vi "ControlSubMIMO.vi"(0 "AxisForceSample":dbl[](array[numeric]), 1 "Command":dbl[](array[numeric]), 3 "Angel":bool[](array[boolean]), 4 "AngleSample":dbl[](array[numeric]), 5 "TorqueSample":dbl[](array[numeric]), 6 "Torque":bool[](array[boolean]), 8 "syn-error":dbl[](array[numeric]), 11 "ChannelSetArray":T1[](array[typedef]) {"Enable" items=["不使能", "使能"]; "Wave" items=["0指令", "正弦波", "方波", "三角波", "常值", "波形数据", "白噪声", "正弦扫频", "梯度加载", "VMIC"]; "ChannelType" items=["标准波形跟踪"=1, "扫频测试"=2, "消除多余力"=3, "梯度加载"=4, "载荷谱跟踪"=5, "模拟输入跟踪"=9]; "ChannelStatus" items=["通道关", "位置通道", "加载通道"]}, 12 "dt":dbl) -> (14 "ControlOutput":dbl[](array[numeric]))   [LabVIEW 2020]
uses:
  ChannelCommand.ctl
  Control 1.ctl
  WaveType.ctl
  MoterEnable.ctl
panel:
  in  "ControlPara":dbl[][](array[numeric])
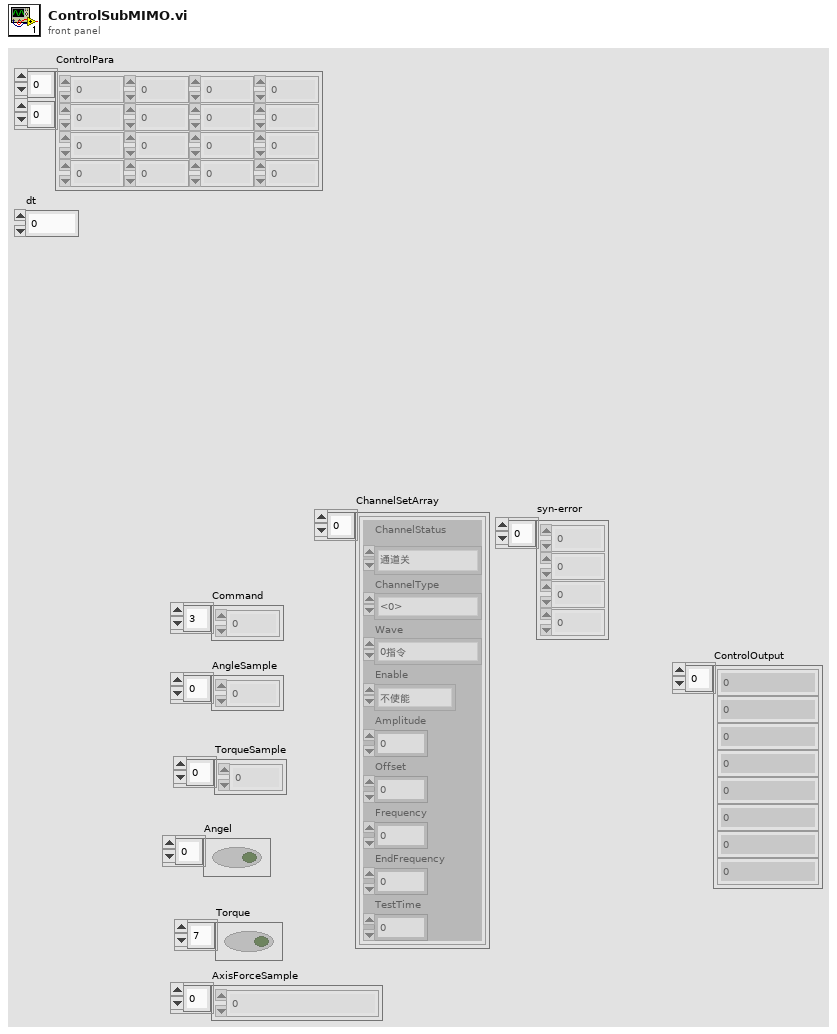
[diagram p1: front panel]
types:
  T1 = typedef "ChannelCommand.ctl" = cluster{"ChannelStatus":T2, "ChannelType":i32, "Wave":T3, "Enable":T4, "Amplitude":dbl, "Offset":dbl, "Frequency":dbl, "EndFrequency":dbl, "TestTime":dbl}
  T2 = typedef "Control 1.ctl" = i32
  T3 = typedef "WaveType.ctl" = i32
  T4 = typedef "MoterEnable.ctl" = u16
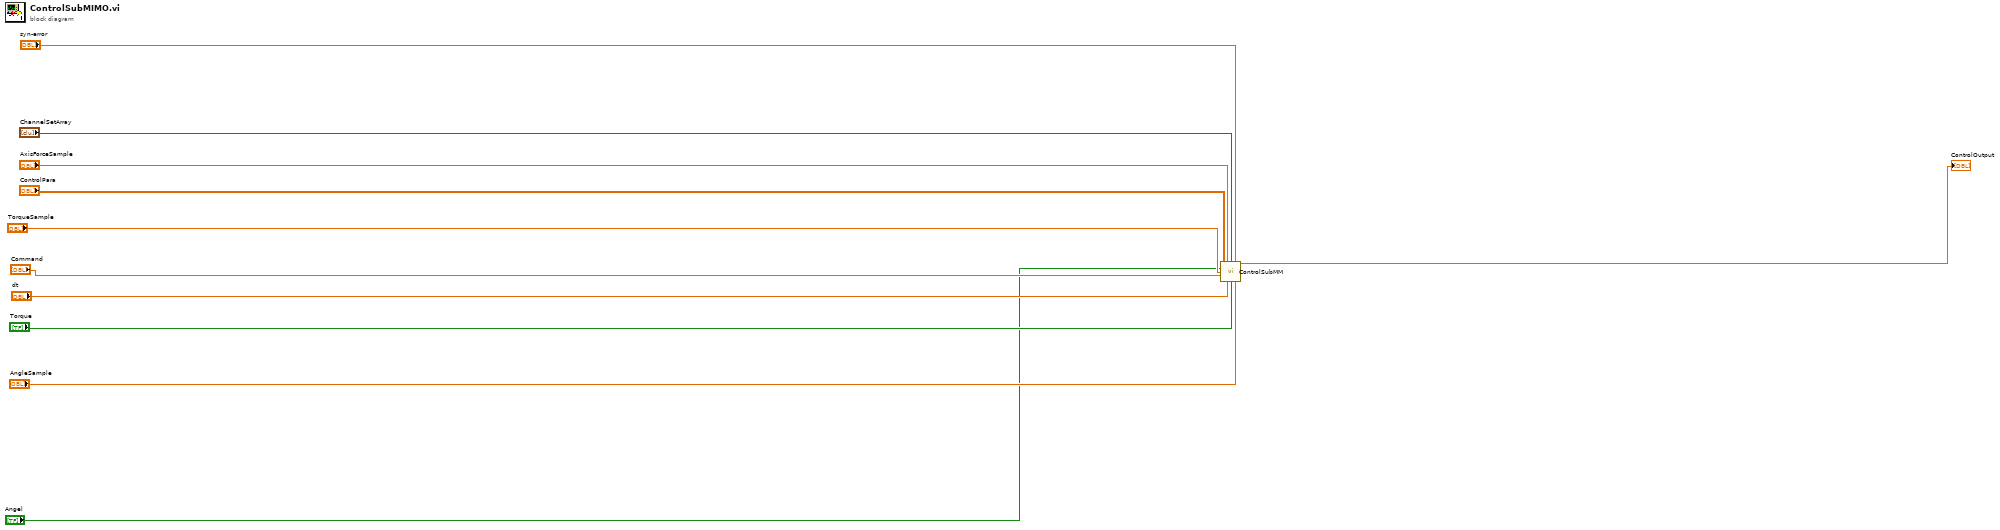
[diagram p0: block diagram]
diagram:
  n1 = call "ControlSubMM.vi"("ControlPara"="ControlPara", "AxisForceSample"="AxisForceSample", "ChannelSetArray"="ChannelSetArray", "syn-error"="syn-error", "Angel"="Angel", "TorqueSample"="TorqueSample", "Command"="Command", "dt"="dt", "Torque"="Torque", "AngleSample"="AngleSample") -> ("数组"=→"ControlOutput":dbl[])  [unwired: 5 in]
